vi "Send Updated Command Status.vi"(7 "Message Priority (Normal)":T3=enum."Normal", 8 "error in (no error)":errorcluster, 10 "Command Status":T1, 11 "Message Enqueuer":refnum<class "Message Enqueuer.lvclass">) -> (0 "error out":errorcluster, 3 "Message Enqueuer out":refnum<class "Message Enqueuer.lvclass">)   [LabVIEW 2014, in "Robot Actor Framework.lvlib" / "System Actor.lvlib" / "Updated Command Status Msg.lvclass"]
doc: "This VI sends the message to an actor."
uses:
  Updated Command Status Msg.lvclass
  <vilib>/ActorFramework/Message Enqueuer/Message Enqueuer.lvclass
  <vilib>/ActorFramework/Message Enqueuer/Message Priority.ctl
  Command Actor/Command Actor Class/Command State.ctl
  Command Actor/Command Actor Class/Command States.ctl
  Updated Command Status Msg.lvclass/Updated Command Status Msg.ctl
  <vilib>/ActorFramework/Message Enqueuer/Message Enqueuer.lvclass/Message Enqueuer.ctl
  <vilib>/ActorFramework/Message Priority Queue/Priority Enqueue.vi
  Command Actor/Command Actor Class/Command Actor.lvclass
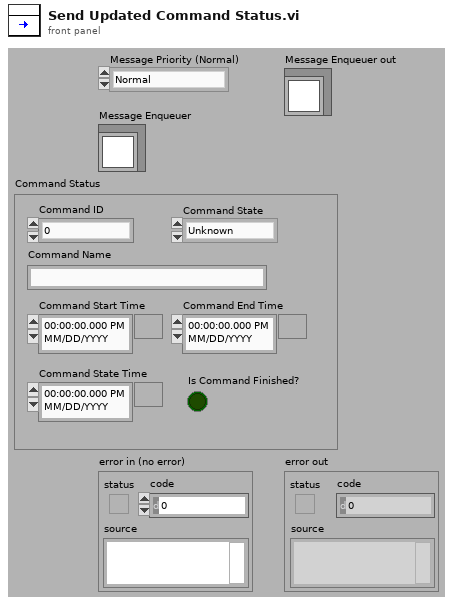
[diagram p1: front panel]
types:
  T1 = typedef "Robot Actor Framework.lvlib/Command Actor.lvlib/Command Actor.lvclass/Command State.ctl" = cluster{"Command Name":string, "Command Start Time":timestamp, "Command End Time":timestamp, "Is Command Finished?":bool, "Command ID":u32, "Command State":T2, "Command State Time":timestamp}
  T2 = typedef "Robot Actor Framework.lvlib/Command Actor.lvlib/Command Actor.lvclass/Command States.ctl" = enum16{"Unknown", "Started", "Stopped", "Finished"}
  T3 = typedef "Actor Framework.lvlib/Message Enqueuer.lvclass/Message Priority.ctl" = enum16{"Low", "Normal", "High"}
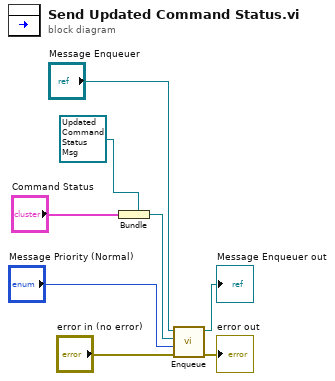
[diagram p0: block diagram]
diagram:
  n1 = Bundle(cluster=refnum<class "Updated Command Status Msg.lvclass"> refnum ("Object"), "Command Status") -> (w4:refnum<class "Updated Command Status Msg.lvclass">)
  n2 = call <vilib>:"Enqueue.vi"("error in (no error)"="error in (no error)", "Message Priority (Normal)"="Message Priority (Normal)", "Message"=w4, "Message Enqueuer in"="Message Enqueuer") -> ("error out"=→"error out":errorcluster, "Message Enqueuer out"=→"Message Enqueuer out":refnum<class "Message Enqueuer.lvclass">)  [unwired: 6 in]
